vi "lsl resolve all.vi"(8 "error in (no error)":errorcluster, 9 "wait_time":dbl) -> (0 "error out":errorcluster, 2 "function return":i32, 3 "Buffer Out":u64[](array[numeric]))   [LabVIEW 2018, in "liblsl-LabVIEW.lvlib"]
doc: "extern LIBLSL_C_API int32_t lsl_resolve_all(lsl_streaminfo *buffer, uint32_t buffer_elements, double wait_time);"
uses:
  <userlib>/liblsl-LabVIEW/liblsl-LabVIEW.lvlib
  <userlib>/liblsl-LabVIEW/liblsl64.dll
panel:
  in  "Buffer Element":u64
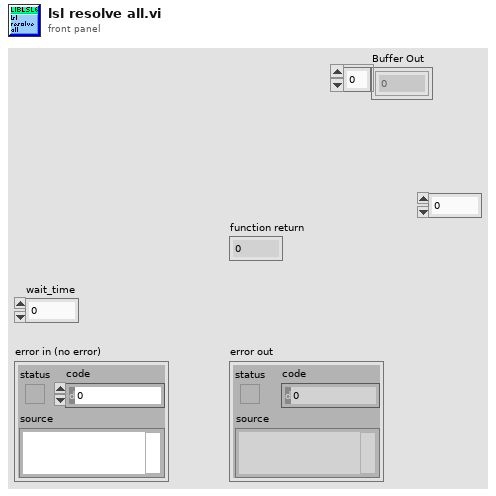
[diagram p1: front panel]
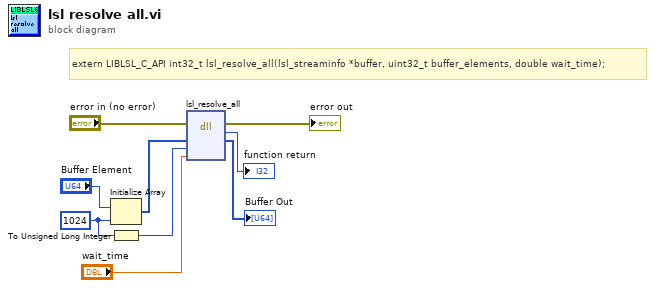
[diagram p0: block diagram]
diagram:
  w1 = 1024 ("dimension size")
  # "extern LIBLSL_C_API int32_t lsl_resolve_all(lsl_streaminfo *buffer, uint32_t buffer_elements, double wait_time);"
  n1 = Initialize Array("Buffer Element", w1) -> (w4:u64[])
  n2 = To Unsigned Long Integer(number=w1) -> (unsigned 32bit integer=w2:u32)
  n3 = dll-call lib="C:/Program Files/National Instruments/LabVIEW 2018/user.lib/liblsl-LabVIEW/liblsl64.*" fn="lsl_resolve_all"(error in="error in (no error)", "buffer"=w4, "buffer_elements"=w2, "wait_time"="wait_time") -> (error out=→"error out":errorcluster, "return type"=→"function return":i32, "buffer"=→"Buffer Out":u64[])  [unwired: 4 in, 1 out]
